vi "www template.vi"(5 "ENV":T1, 6 "User Information":T2, 7 "Template (\"\")":string, 8 "error in (no error)":errorcluster, 9 "Replaceable Keys (empty)":T1, 10 "HTTP Header In (\"\")":string, 11 "Connection Refnum":T3) -> (0 "error out":errorcluster, 1 "HTTP Template Content":string, 2 "HTTP Header Out":string, 3 "Connection Refnum":T3)   [LabVIEW 2011]
uses:
  Addons/internet/utils/keyedarr.llb/Keyed Array.ctl
  SI.LIB/ODBC/SQL Controls/Connection Refnum.ctl
  server/database/Users/User Record.ctl
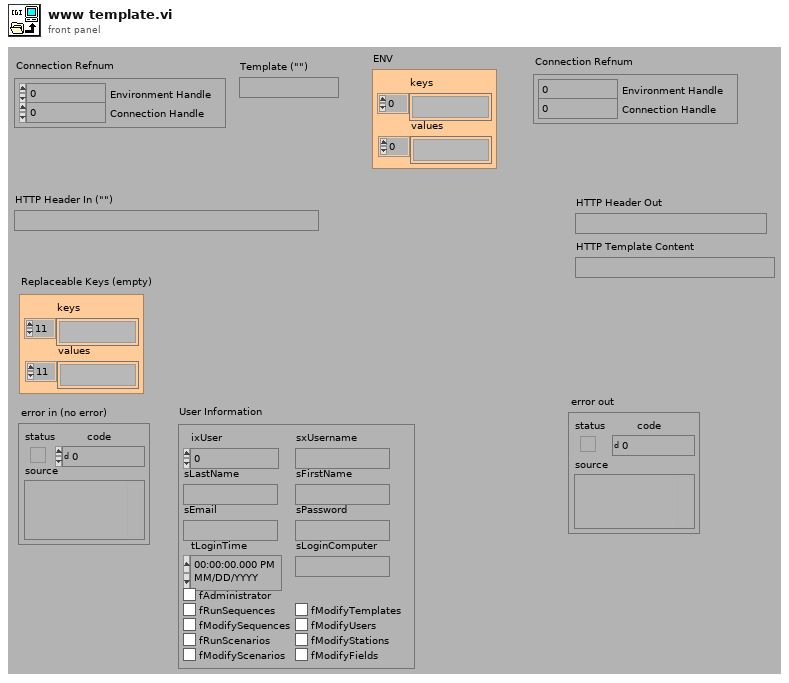
[diagram p1: front panel]
types:
  T1 = typedef "Keyed Array.ctl" = cluster{"keys":string[], "values":string[]}
  T2 = typedef "User Record.ctl" = cluster{"ixUser":i32, "sxUsername":string, "sLastName":string, "sFirstName":string, "sEmail":string, "sPassword":string, "tLoginTime":timestamp, "sLoginComputer":string, "fAdministrator":bool, "fRunSequences":bool, "fModifySequences":bool, "fRunScenarios":bool, "fModifyScenarios":bool, "fModifyTemplates":bool, "fModifyUsers":bool, "fModifyStations":bool, "fModifyFields":bool}
  T3 = typedef "Connection Refnum.ctl" = cluster{"Environment Handle":i32, "Connection Handle":i32}
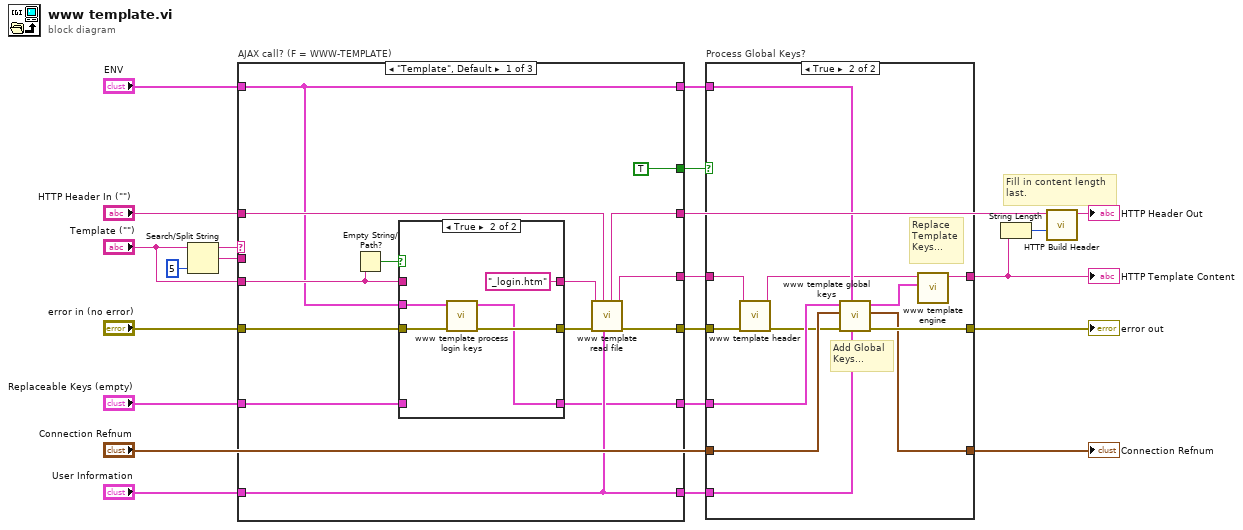
[diagram p0: block diagram]
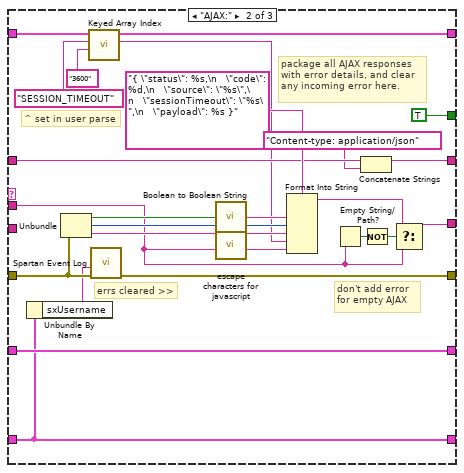
[diagram p4: hidden frame]
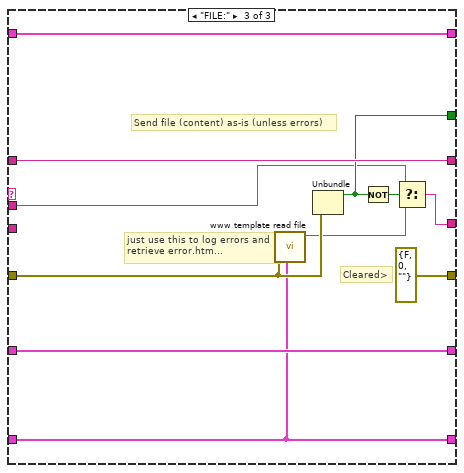
[diagram p5: hidden frame]
diagram:
  # "Fill in content length\nlast."
  n1 = Search/Split String(string="Template (\"\")", offset (0)=5) -> (substring before match=w9:string, match + rest of string=w8:string)  [unwired: 2 out]
  n2 = case "AJAX call? (F = WWW-TEMPLATE)" shown="\"Template\", Default" w9 {
    tunnel: [w32 w50 errorcluster {"status"=FALSE, "code"=0, "source"=""} ("error out")] -> w16
    tunnel: "error in (no error)" -> [w24 w57 w77]
    tunnel: "HTTP Header In (\"\")" -> [w36 w55 w80]
    tunnel: [w35 w54 w80] -> w13
    tunnel: [w33 w61 w79] -> w12
    tunnel: "User Information" -> [w31 w51 w70]
    tunnel: w8 -> [_ w59 w73]
    tunnel: [TRUE TRUE w78] -> w7
    tunnel: "Template (\"\")" -> [w29 _ _]
    tunnel: "ENV" -> [w25 w49 w72]
    tunnel: [w25 w48 w72] -> w4
    tunnel: "Replaceable Keys (empty)" -> [w27 w52 w71]
    tunnel: [w26 w52 w71] -> w2
    tunnel: [w31 w51 w70] -> w1
    frame "Template", Default {
      n3 = Empty String/Path?(string/path=w29) -> (empty?=w30:bool)
      n4 = case shown="True" w30 {
        tunnel: w29 -> [w39 _]
        tunnel: [w39 "_login.htm" ("Template (\"\")")] -> w28
        tunnel: w27 -> [w38 _]
        tunnel: [w38 w40] -> w26
        tunnel: w25 -> [_ w41]
        tunnel: w24 -> [w37 w43]
        tunnel: [w37 w42] -> w23
        frame False {
        }
        frame True {
          n5 = call "www template process login keys.vi"("error in (no error)"=w43, "ENV"=w41) -> ("error out"=w42:errorcluster, "Login Keys"=w40:T1)  [unwired: 8 out]
        }
      }
      n6 = call "www template read file.vi"("User Information"=w31, "HTTP Header (\"\")"=w36, "error in (no error)"=w23, "Template File (\"\")"=w28) -> ("error out"=w32:errorcluster, "Page HTML"=w33:string, "new HTTP Header"=w35:string)  [unwired: 5 out]
    }
    frame "AJAX:" {
      # "^ set in user parse"
      # "errs cleared >>"
      # "don't add error\nfor empty AJAX"
      # "package all AJAX responses\nwith error details, and clear\nany incoming error here."
      n7 = Unbundle By Name(w51) -> ("sxUsername"=w56:string)
      n8 = Unbundle(w57) -> ("status"=w67:bool, "code"=w66:i32, "source"=w65:string)
      n9 = call "Keyed Array Index.vi"("default value"="3600", "key"="SESSION_TIMEOUT", "array in"=w49) -> ("value"=w47:string, "duplicate array"=w48:T1)  [unwired: 1 in, 2 out]
      n10 = call "Spartan Event Log.vi"("error in (no error)"=w57, "username (\"\")"=w56) -> ("error out"=w50:errorcluster)  [unwired: 3 in, 3 out]
      n11 = call "Boolean to Boolean String.vi"("Boolean"=w67) -> ("Boolean string"=w68:string)  [unwired: 1 in]
      n12 = call "escape characters for javascript.vi"("String (\"\")"=w65) -> ("escaped String"=w64:string)  [unwired: 4 out]
      n13 = Format Into String(format string="{ \"status\": %s,\n   \"code\": %d,\n   \"source\": \"%s\",\n   \"sessionTimeout\": \"%s\",\n   \"payload\": %s }", w68, w66, w64, w47, w59) -> (resulting string=w62:string)  [unwired: 2 in, 1 out]
      n14 = Empty String/Path?(string/path=w59) -> (empty?=w63:bool)
      n15 = Concatenate Strings(w55, "Content-type: application/json") -> (w54:string)
      n16 = Not(x=w63) -> (.not. x?=w60:bool)
      n17 = Select(t=w62, s=w60, f=w59) -> (s? t:f=w61:string)
    }
    frame "FILE:" {
      # "Cleared>"
      # "just use this to log errors and\nretrieve error.htm..."
      # "Send file (content) as-is (unless errors)"
      n18 = call "www template read file.vi"("User Information"=w70, "error in (no error)"=w77) -> ("Page HTML"=w75:string)  [unwired: 2 in, 7 out]
      n19 = Unbundle(w77) -> ("status"=w78:bool)  [unwired: 2 out]
      n20 = Not(x=w78) -> (.not. x?=w76:bool)
      n21 = Select(t=w73, s=w76, f=w75) -> (s? t:f=w79:string)
    }
  }
  n22 = case "Process Global Keys?" shown="True" w7 {
    tunnel: [w82 w95] -> w22
    tunnel: [w83 w94] -> w21
    tunnel: w2 -> [_ w93]
    tunnel: "Connection Refnum" -> [w81 w92]
    tunnel: [w81 w91] -> w17
    tunnel: w16 -> [w82 w87]
    tunnel: w12 -> [w83 w85]
    tunnel: w1 -> [_ w89]
    tunnel: w4 -> [_ w88]
    frame False {
    }
    frame True {
      # "Replace\nTemplate\nKeys..."
      # "Add Global\nKeys..."
      n23 = call "www template header.vi"("error in (no error)"=w87, "Template Content (\"\")"=w85) -> ("error out"=w86:errorcluster, "Template Content"=w84:string)  [unwired: 3 in, 5 out]
      n24 = call "www template global keys.vi"("Current User"=w89, "ENV"=w88, "error in (no error)"=w86, "Connection Refnum"=w92, "Template Keys In (empty)"=w93) -> ("error out"=w95:errorcluster, "Connection Refnum"=w91:T3, "new Template Keys"=w90:T1)  [unwired: 4 out]
      n25 = call "www template engine.vi"("Template Dictionary (empty)"=w90, "Template String (\"\")"=w84) -> ("Template String out"=w94:string)  [unwired: 1 in, 8 out]
    }
  }
  "error out" <- w22
  "HTTP Template Content" <- w21
  "Connection Refnum" <- w17
  n26 = String Length(string=w21) -> (length=w19:i32)
  n27 = call "HTTP Build Header.vi"("content length (-1)"=w19, "header"=w13) -> ("full header"=→"HTTP Header Out":string)  [unwired: 2 in, 7 out]
